vi "USB Device History Cleanup.vi"() -> ()   [LabVIEW 2018]
panel:
  in  "Main Tab":enum32{"Control", "Maint"}(tab)
  in  "Abort":bool
  out "Busy":bool
  out "StdOut":string
  out "Cmd":string
  out "Search ID":string
  out "Total":i32
  out "Progress":dbl(slide) scale=0.0..1.0
  in  "Remove USB History":bool
  in  "PID":string
  in  "VID":string="28DE"
  out "Completed":i32
  out "Device List":string[][](array[string])
  out "Errors":errorcluster
  # "(Required)"
  # "(Optional)"
  # "DevCon"
  # "!This app must be run as Adminsitrator to have permissions to edit the registry."
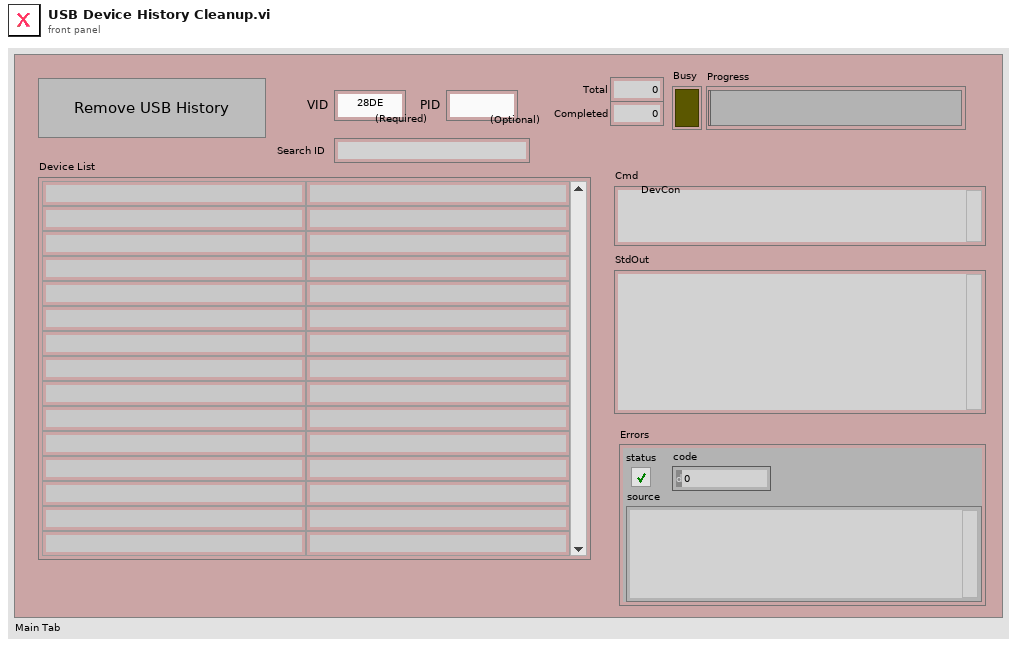
[diagram p1: front panel]
types:
  T1 = enum32{"invalid app kind", "Development System", "Run Time System", "Student Edition", "Embedded LabVIEW", "Evaluation", "Custom"}
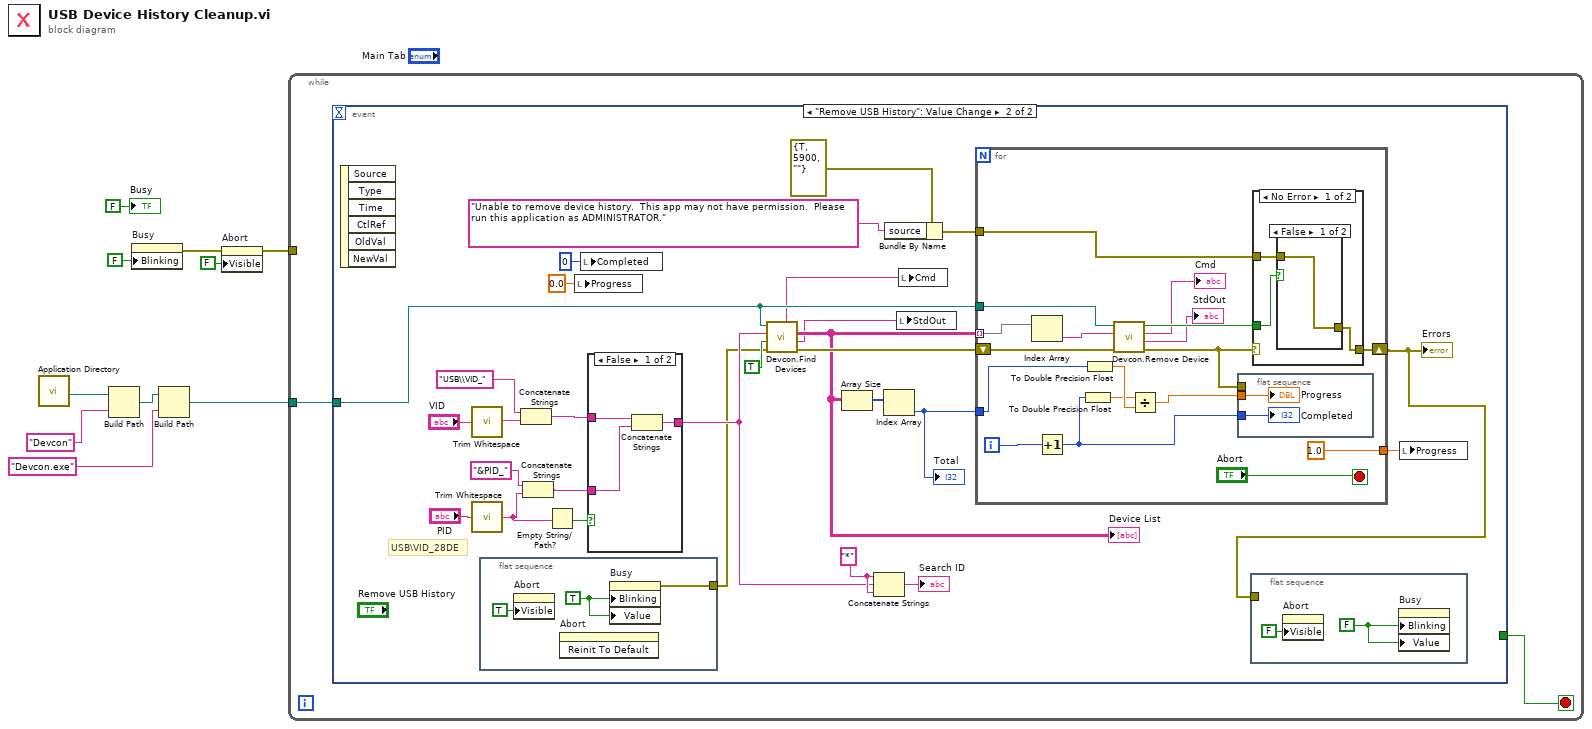
[diagram p0: block diagram]
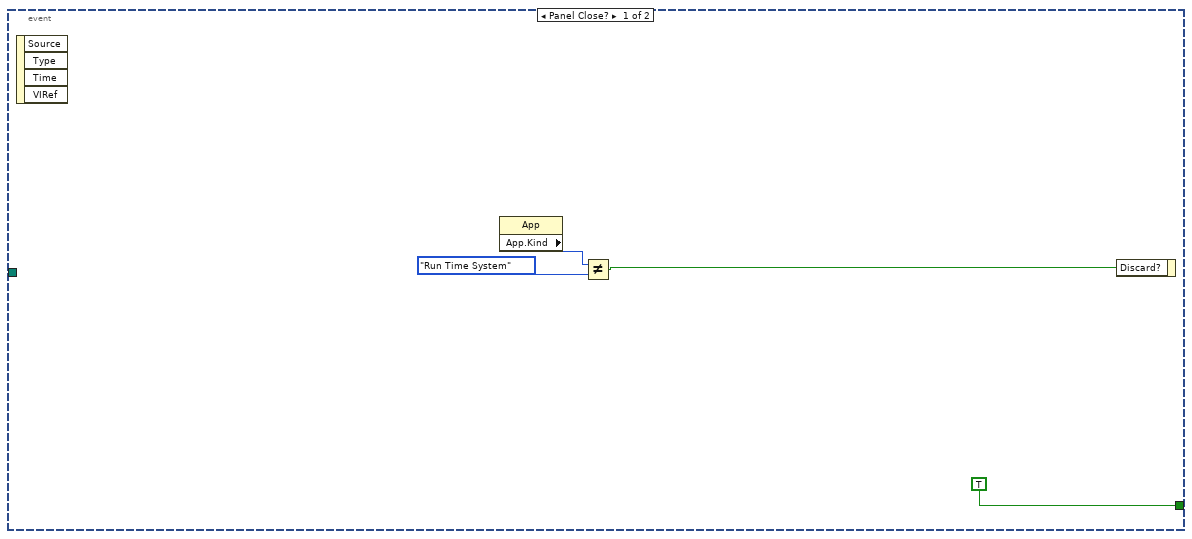
[diagram p2: hidden frame]
diagram:
  n1 = call <vilib>:"Application Directory.vi"() -> ("Application Directory"=w9:path)
  n2 = Build Path(base path=w9, name or relative path="Devcon") -> (appended path=w10:path)
  n3 = property on="Busy" class="Bool (strict)"("Blinking"=FALSE) -> (error out=w2:errorcluster)  [unwired: 2 in, 1 out]
  n4 = Build Path(base path=w10, name or relative path="Devcon.exe") -> (appended path=w6:path)
  n5 = property on="Abort" class="Bool"(error in=w2, "Visible"=FALSE) -> (error out=w1:errorcluster)  [unwired: 1 in, 1 out]
  n6 = while {
    tunnel: w6 -> [w11]
    tunnel: w1 -> [_]
    stop <- w12 stop-if-true
    n7 = event shown="[1] \"Remove USB History\": Value Change" {
      selector: _ -> [_ _]
      dyn-events: _ -> [_ _]
      timeout: _ -> [_ _]
      tunnel: [TRUE _] -> w12
      tunnel: w11 -> [_ w42]
      event Panel Close? {
        n8 = event-data() -> ()  [unwired: 1 in, 4 out]
        n9 = property class="App"() -> ("App.Kind"=w15:T1)  [unwired: 2 in, 2 out]
        n10 = Not Equal?(x=w15, y=T1."Run Time System") -> (x != y?=w13:bool)
        n11 = event-data("Discard?"=w13) -> ()  [unwired: 1 in, 1 out]
      }
      event "Remove USB History": Value Change {
        w34 = "*"
        # "USB\\VID_28DE"
        n12 = event-data() -> ()  [unwired: 1 in, 6 out]
        n13 = call <vilib>:"Trim Whitespace.vi"("string"="VID") -> ("trimmed string"=w31:string)  [unwired: 1 in]
        n14 = call <vilib>:"Trim Whitespace.vi"("string"="PID") -> ("trimmed string"=w27:string)  [unwired: 1 in]
        n15 = flat-sequence {
          tunnel: [w46] -> w20
          frame #0 {
            w47 = TRUE ("Blinking")
            n16 = property on="Abort" class="Bool"("Visible"=TRUE) -> ()  [unwired: 2 in, 2 out]
            n17 = invoke on="Abort" class="Bool" method="Reinit To Default"() -> ()  [unwired: 3 in, 3 out]
            n18 = property on="Busy" class="Bool (strict)"("Blinking"=w47, "Value"=w47) -> (error out=w46:errorcluster)  [unwired: 2 in, 1 out]
          }
        }
        n19 = Concatenate Strings("USB\\VID_", w31) -> (w29:string)
        n20 = Concatenate Strings("&PID_", w27) -> (w26:string)
        n21 = Empty String/Path?(string/path=w27) -> (empty?=w36:bool)
        n22 = local write "Progress"(0.0 ("Progress")) -> ()
        n23 = local write "Completed"(0 ("Completed")) -> ()
        n24 = case shown="False" w36 {
          tunnel: w26 -> [w51 _]
          tunnel: w29 -> [w52 w53]
          tunnel: [w50 w53] -> w33
          frame False {
            n25 = Concatenate Strings(w52, w51) -> (w50:string)
          }
          frame True {
          }
        }
        n26 = call "Devcon.Find Devices.vi"("error in (no error)"=w20, "State(Present(F), All(T))"=TRUE, "DeviceID"=w33, "DevconEXE"=w42) -> ("error out"=w44:errorcluster, "StdOut"=w22:string, "Device List"=w41:string[][], "Cmd"=w21:string)  [unwired: 3 in, 1 out]
        "Device List" <- w41
        n27 = Array Size(array=w41) -> (size(s)=w40:i32[])
        n28 = Concatenate Strings(w34, w33, w34) -> (→"Search ID":string)
        n29 = Index Array(array=w40) -> (element=w38:i32)  [unwired: 1 in]
        "Total" <- w38
        n30 = Bundle By Name(cluster=errorcluster {"status"=TRUE, "code"=5900, "source"=""} ("error constant"), "source"="Unable to remove device history.  This app may not have permission.  Please run this application as ADMINISTRATOR.") -> (w23:errorcluster)
        n31 = local write "StdOut"(w22) -> ()
        n32 = local write "Cmd"(w21) -> ()
        n33 = for {
          tunnel: w41 -> [w70] mode=indexing
          tunnel: w42 -> [w71]
          shift-right: [w62] -> w19
          shift-left: w44 -> [w68]
          tunnel: w38 -> [w67]
          tunnel: [1.0] -> w39
          tunnel: w23 -> [w60]
          i -> [w56]
          stop <- "Abort" stop-if-true
          n34 = Index Array(array=w70) -> (element=w69:string)  [unwired: 1 in]
          n35 = Increment(x=w56) -> (x+1=w55:i32)
          n36 = To Double Precision Float(number=w55) -> (double precision float=w65:dbl)
          n37 = To Double Precision Float(number=w67) -> (double precision float=w66:dbl)
          n38 = call "Devcon.Remove Device.vi"("error in (no error)"=w68, "DeviceID"=w69, "DevconEXE"=w71) -> ("error out"=w54:errorcluster, "StdOut"=→"StdOut":string, "Cmd"=→"Cmd":string, "Success"=w61:bool)  [unwired: 5 in]
          n39 = Divide(x=w65, y=w66) -> (x/y=w64:dbl)
          n40 = flat-sequence {
            tunnel: w64 -> [w73]
            tunnel: w55 -> [w72]
            tunnel: w54 -> [_]
            frame #0 {
              "Completed" <- w72
              "Progress" <- w73
            }
          }
          n41 = case shown="No Error" w54 {
            selector: w54 -> [_ w78]
            tunnel: [w75 w78] -> w62
            tunnel: w61 -> [w76 _]
            tunnel: w60 -> [w74 _]
            frame No Error {
              n42 = case shown="False" w76 {
                tunnel: [w77 _] -> w75
                tunnel: w74 -> [w77 _]
                frame False {
                }
                frame True {
                }
              }
            }
            frame Error {
            }
          }
        }
        "Errors" <- w19
        n43 = flat-sequence {
          tunnel: w19 -> [_]
          frame #0 {
            w49 = FALSE ("Blinking")
            n44 = property on="Abort" class="Bool"("Visible"=FALSE) -> ()  [unwired: 2 in, 2 out]
            n45 = property on="Busy" class="Bool (strict)"("Blinking"=w49, "Value"=w49) -> ()  [unwired: 2 in, 2 out]
          }
        }
        n46 = local write "Progress"(w39) -> ()
      }
    }
  }
  "Busy" <- FALSE ("Busy")
